vi "Convert Absolute to Relative Path if Executable.vi"(8 "error in (no error)":errorcluster, 11 "Absolute Path":path) -> (0 "error out":errorcluster, 2 "Relative Path?":bool, 3 "Result Path":path)   [LabVIEW 2020, in "RxnRover.lvlib" / "File IO.lvlib"]
doc: "Converts an absolute path to a relative path if the application is being executed as an executable. The absolute path is retained if a development environment is being used."
uses:
  File IO.lvlib
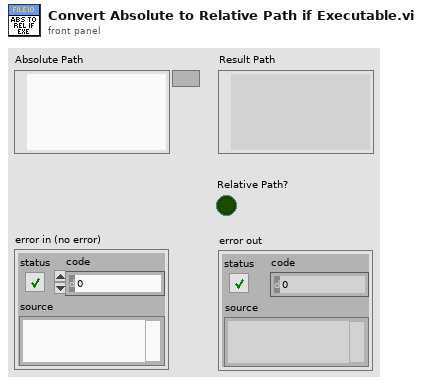
[diagram p1: front panel]
types:
  T1 = enum32{"invalid app kind", "Development System", "Run Time System", "Student Edition", "Embedded LabVIEW", "Evaluation", "Custom"}
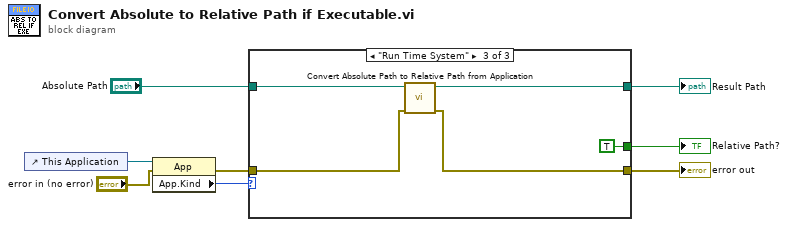
[diagram p0: block diagram]
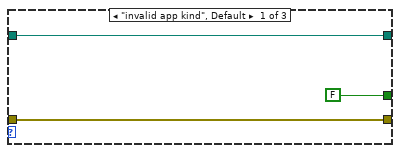
[diagram p2: hidden frame]
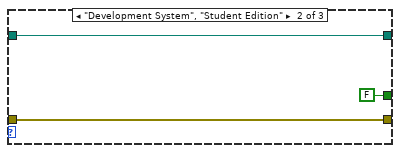
[diagram p3: hidden frame]
diagram:
  n1 = control-ref of="This Application"() -> (w8:refnum<vi>)
  n2 = property class="App"(reference=w8, error in="error in (no error)") -> (error out=w4:errorcluster, "App.Kind"=w6:T1)  [unwired: 1 out]
  n3 = case shown="\"Run Time System\"" w6 {
    tunnel: "Absolute Path" -> [w9 w14 w19]
    tunnel: [w9 w14 w15] -> w1
    tunnel: w4 -> [w10 w12 w18]
    tunnel: [w10 w12 w17] -> w3
    tunnel: [FALSE FALSE TRUE] -> w2
    frame "invalid app kind", Default {
    }
    frame "Development System", "Student Edition" {
    }
    frame "Run Time System" {
      n4 = call "Convert Absolute Path to Relative Path from Application.vi"("error in (no error)"=w18, "Absolute Path"=w19) -> ("error out"=w17:errorcluster, "Relative Path"=w15:path)  [unwired: 8 in]
    }
  }
  "error out" <- w3
  "Result Path" <- w1
  "Relative Path?" <- w2
